vi "Condition Type.vi"(11 "Condition Config in":refnum<class "Condition Config.lvclass">) -> (2 "Condition Type":string)   [LabVIEW 2020, in "VolatusSeqConfig.lvlib" / "Condition Config.lvclass"]
uses:
  Condition Config.lvclass
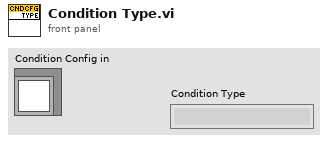
[diagram p1: front panel]
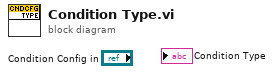
[diagram p0: block diagram]
diagram:
